vi "Write start time.vi"(8 "error in":errorcluster, 10 "start time":timestamp, 11 "timing source in":refnum<class "absolute usec timing source.lvclass">) -> (0 "error out":errorcluster, 3 "timing source out":refnum<class "absolute usec timing source.lvclass">)   [LabVIEW 2013, in "absolute usec timing source.lvclass"]
doc: "Sets the start time of an absolute timing source"
uses:
  absolute usec timing source.lvclass
  absolute usec timing source.lvclass/absolute usec timing source.ctl
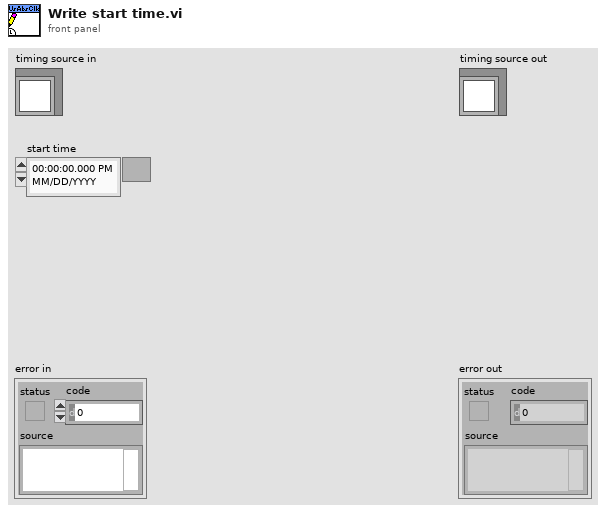
[diagram p1: front panel]
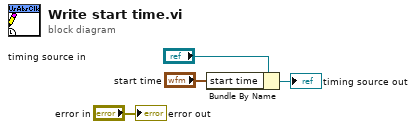
[diagram p0: block diagram]
diagram:
  n1 = Bundle By Name(cluster="timing source in", "start time"="start time") -> (→"timing source out":refnum<class "absolute usec timing source.lvclass">)
  "error out" <- "error in"
